vi "Generate RPC Client Methods.vi"(7 "RPC Method Parameters":T1[](array[typedef]), 8 "error in (no error)":errorcluster, 11 "Server class in":refnum<vi>) -> (0 "error out":errorcluster, 3 "Server class out":refnum<vi>)   [LabVIEW 2019, in "gRPC Scripting Tools.lvlib"]
uses:
  gRPC Scripting Tools.lvlib
  TypeDefs/RPC Method Parameters.ctl
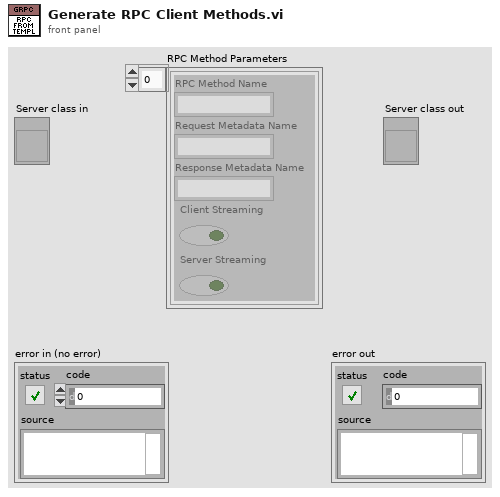
[diagram p1: front panel]
types:
  T1 = typedef "gRPC Scripting Tools.lvlib/RPC Method Parameters.ctl" = cluster{"RPC Method Name":string, "Request Metadata Name":string, "Response Metadata Name":string, "Client Streaming":bool, "Server Streaming":bool}
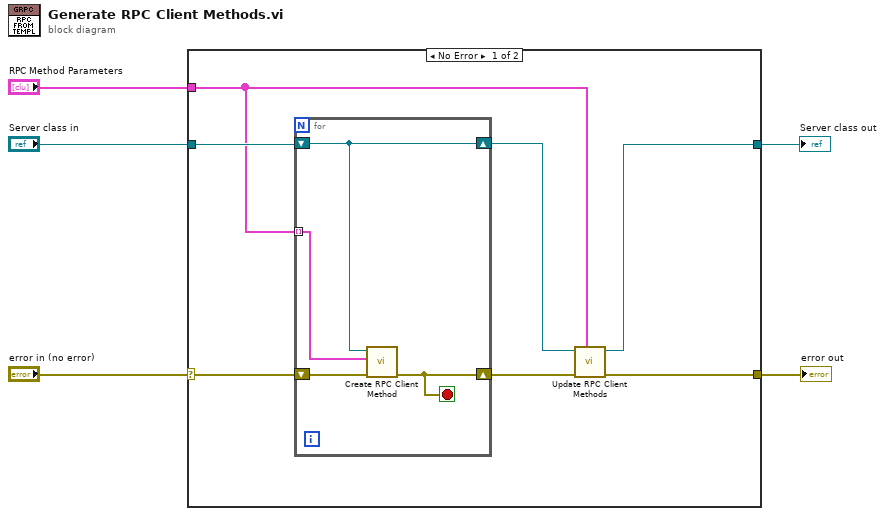
[diagram p0: block diagram]
diagram:
  n1 = case shown="No Error" "error in (no error)" {
    selector: "error in (no error)" -> [w12 w18]
    tunnel: [w7 w18] -> w5
    tunnel: "Server class in" -> [w11 w17]
    tunnel: [w6 w17] -> w2
    tunnel: "RPC Method Parameters" -> [w9 _]
    frame No Error {
      n2 = for {
        tunnel: w9 -> [w13] mode=indexing
        shift-right: [w14] -> w10
        shift-left: w12 -> [w16]
        shift-right: [w15] -> w8
        shift-left: w11 -> [w15]
        stop <- w14 stop-if-true
        n3 = call "Create RPC Client Method.vi"("error in (no error)"=w16, "RPC Method Parameters"=w13, "Server class in"=w15) -> ("error out"=w14:errorcluster)  [unwired: 6 in, 2 out]
      }
      n4 = call "Update RPC Client Methods.vi"("RPC Method Parameters"=w9, "error in (no error)"=w10, "Server class in"=w8) -> ("error out"=w7:errorcluster, "Server class out"=w6:refnum<vi>)  [unwired: 7 in]
    }
    frame Error {
    }
  }
  "error out" <- w5
  "Server class out" <- w2
